vi "randomize.vi"(1 "Input array":dbl[](array[numeric])) -> (0 "Output array":dbl[](array[numeric]))   [LabVIEW 2015]
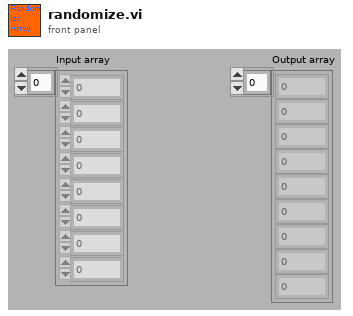
[diagram p1: front panel]
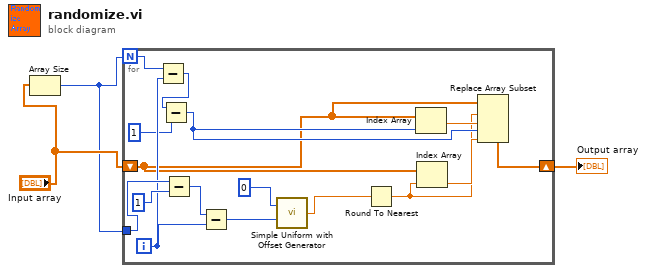
[diagram p0: block diagram]
diagram:
  n1 = Array Size(array="Input array") -> (size(s)=w1:i32)
  n2 = for {
    N: w1 -> [w16]
    shift-right: [w12] -> w2
    shift-left: "Input array" -> [w4]
    tunnel: w1 -> [w19]
    i -> [w15]
    n3 = Subtract(x=w16, y=w15) -> (x-y=w10:i32)
    n4 = Subtract(x=w10, y=1) -> (x-y=w11:i32)
    n5 = Subtract(x=w19, y=1) -> (x-y=w17:i32)
    n6 = Subtract(x=w17, y=w15) -> (x-y=w8:i32)
    n7 = call "Simple Uniform with Offset Generator.vi"("a"=w8, "b"=0) -> ("X"=w6:dbl)
    n8 = Round To Nearest(number=w6) -> (nearest integer value=w5:dbl)
    n9 = Index Array(array=w4, index=w11) -> (element=w13:dbl)
    n10 = Index Array(array=w4, index=w5) -> (element=w14:dbl)
    n11 = Replace Array Subset(array=w4, new element #1=w13, index #1=w5, new element #2=w14, index #2=w11) -> (w12:dbl[])
  }
  "Output array" <- w2
